vi "Register_Command_Pointer.vi"(8 "error in (no error)":errorcluster, 10 "Strict-Typed VI Refnum":refnum<vi>, 11 "Name":string) -> (0 "error out":errorcluster)   [LabVIEW 2012]
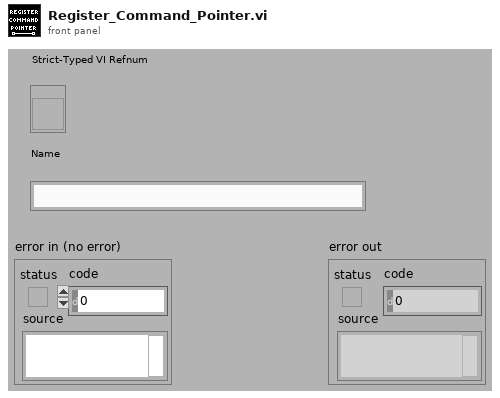
[diagram p1: front panel]
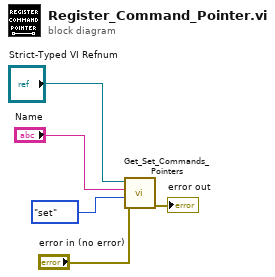
[diagram p0: block diagram]
diagram:
  n1 = call "Get_Set_Commands_Pointers.vi"("error in (no error)"="error in (no error)", "menu"=enum16{"set", "get", "delete"}."set", "refnum name"="Name", "VI Refnum In"="Strict-Typed VI Refnum") -> ("error out"=→"error out":errorcluster)  [unwired: 6 in, 1 out]
